vi "Cross_Correlation.vi"() -> (5 "Plug in titles":string[](array[string]), 7 "Plug in values":string[](array[string]))   [LabVIEW 2012]
uses:
  Globals/Meas_global.vi
panel:
  out "XY Graph":cluster{dbl[], dbl[]}[](graph)
  in  "Time window half width":dbl=3.0
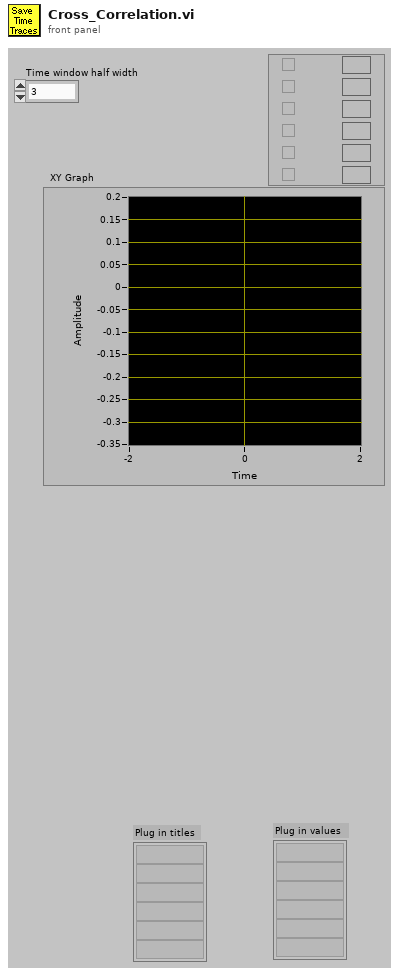
[diagram p1: front panel]
types:
  T1 = typedef "Time_Trace_Cluster.ctl" = cluster{"Weighting":dbl[], "Time (s)":dbl[], "Voltage":dbl[], "Eng Values":dbl[]}
  T2 = typedef "Analysis_info_cluster.ctl" = cluster{"Colour":u32, "Inst type":T3, "Inst name":string, "Symbol":string, "Code name":string, "Extra Info":string, "Inst Array":T4, "Extra Titles":string[], "Extra Values":string[], "U":dbl, "u^2":dbl, "u^3":dbl, "u^4":dbl, "Skew_u":dbl, "Kurt_u":dbl, "Sd Error in Mean":dbl, "% u'/U":dbl, "X":dbl, "Y":dbl, "Z":dbl, "Timescale integral to 25%":dbl, "Sd Error in Variance":dbl, "Calib File":path, "Calib Constants":dbl[], "Output Position":bool, "Full Stats":bool, "Av Sampling Rate":dbl, "Av No of Samples":dbl, "Total Meas Time (s)":dbl, "ADAM Ch Name":string}
  T3 = typedef "Inst_type.ctl" = enum16{"Propeller anemometer", "Raw voltage", "Pressure Transducer", "Pitot-static tube", "Preston tube", "Hot wire", "Cross wire 1", "Cross wire 2", "Generic Linear", "Generic Polynomial", "Generic BackPoly", "Fast FID", "Thermocouple", "Cold wire", "Pulsed Wire", "LDA Vel", "LDA Tran time", "LDA Arr time"}
  T4 = typedef "Instrument_Array.ctl" = enum16{"PWA", "LDA", "Analogue"}
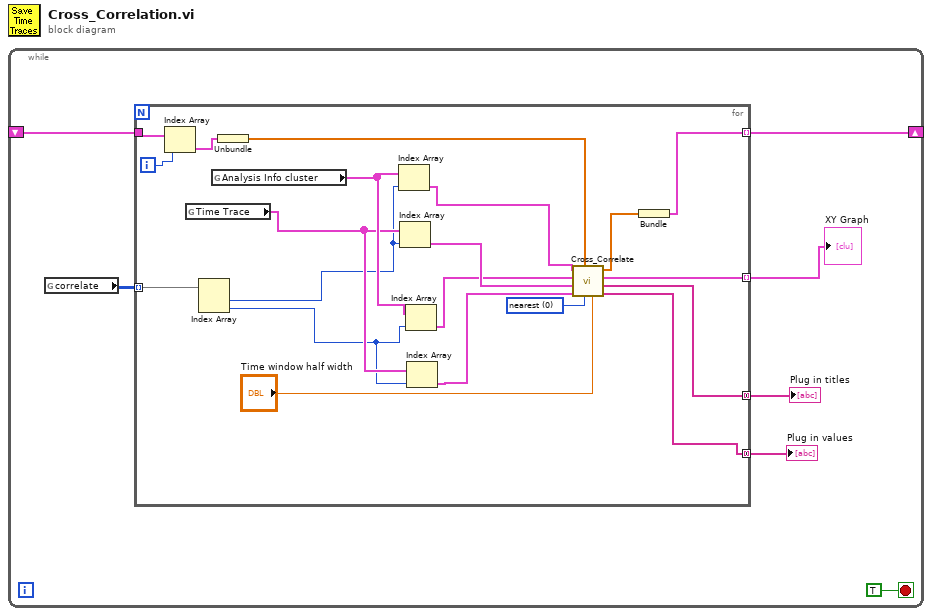
[diagram p0: block diagram]
diagram:
  n1 = while {
    shift-right: [w6] -> _
    shift-left: _ -> [w5]
    stop <- TRUE stop-if-true
    n2 = global read "Meas_global.vi" "correlate"() -> (w7:i32[][])
    n3 = for {
      tunnel: w7 -> [w20] mode=indexing
      tunnel: [w15] -> w6 mode=indexing
      tunnel: w5 -> [w12]
      tunnel: [w8] -> w3 mode=concatenating
      tunnel: [w10] -> w4 mode=indexing
      tunnel: [w9] -> w2 mode=concatenating
      i -> [w13]
      w21 = 0 items=["nearest", "linear", "spline", "cubic Hermite", "Lagrange"] ("interp. method")
      n4 = Index Array(array=w12, index=w13) -> (element=w11:cluster{"Shift output array":dbl[]})
      n5 = global read "Meas_global.vi" "Time Trace"() -> (w26:T1[])
      n6 = Index Array(array=w20) -> (element #1=w19:i32, element #2=w18:i32)  [unwired: 2 in]
      n7 = global read "Meas_global.vi" "Analysis Info cluster"() -> (w27:T2[])
      n8 = Unbundle(w11) -> ("Shift output array"=w14:dbl[])
      n9 = Index Array(array=w27, index=w19) -> (element=w23:T2)
      n10 = Index Array(array=w26, index=w19) -> (element=w25:T1)
      n11 = Index Array(array=w27, index=w18) -> (element=w22:T2)
      n12 = Index Array(array=w26, index=w18) -> (element=w24:T1)
      n13 = call "Cross_Correlate.vi"("Time window half width"="Time window half width", "interp. method"=w21, "Shift input array"=w14, "Time Cluster 2"=w24, "Time Cluster 1"=w25, "Cluster 2"=w22, "Cluster 1"=w23) -> ("Plug In Values"=w8:string[], "Plug In Titles"=w9:string[], "XY Graph"=w10:cluster{dbl[], dbl[]}, "Shift output array"=w16:dbl[])  [unwired: 1 in]
      n14 = Bundle("Shift output array"=w16) -> (w15:cluster{"Shift output array":dbl[]})  [unwired: 1 in]
    }
    "Plug in titles" <- w2
    "Plug in values" <- w3
    "XY Graph" <- w4
  }
